vi "Render Energy.vi"(7 "Renderer":refnum<class "Renderer.lvclass">, 8 "error in (no error)":errorcluster, 11 "Ship in":refnum<class "Ship.lvclass">) -> (0 "error out":errorcluster)   [LabVIEW 2021, in "Ship.lvclass"]
uses:
  Ship.lvclass
  C:/dev/LabVIEW/LabMelee/Source/Application Specific/Element/Element.lvclass
  Renderer/Renderer.lvclass
  Element/Element.lvclass/Element.ctl
  Ship.lvclass/Ship.ctl
  Re-use Libraries/Vector 2D/Vector 2D.lvclass/Vector 2D.ctl
  Re-use Libraries/Vector 2D/Vector 2D.lvclass
  Element/Element.lvclass
  LabSDL2/Source/Libraries/LibSDL2 Wrapper/LibSDL2.lvlib
panel:
  in  "x Offset From Sidebar":i32=180
  in  "y Offset":i32=230
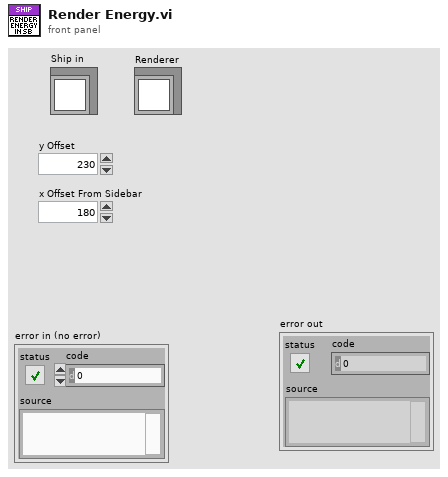
[diagram p1: front panel]
types:
  T1 = typedef "Constants.ctl" = cluster{"Colours":cluster{"OK":u32, "Warning":u32, "Error":u32, "Red":u32, "Green":u32, "Blue":u32, "Yellow":u32, "Health":u32, "Energy":u32}, "System":cluster{"Target Frames Second":dbl, "Windows Size":refnum<class "Vector 2D.lvclass">, "World Size":refnum<class "Vector 2D.lvclass">, "Battle Area Size":refnum<class "Vector 2D.lvclass">, "Sidebar Width":sgl, "SC2 Frame Rate [Seconds/Frame]":sgl, "Sidebar Player 2 Y Offset":sgl}, "Game":cluster{"Maximum Asteroids":i32, "Max Energy":i32, "Max Crew":i32, "Maximum Stars":i32}}
  T2 = typedef "Element.lvclass/Player Type.ctl" = enum16{"Neutral", "Player 1", "Player 2"}
  T3 = typedef "LibSDL2.lvlib/Rectangle.ctl" = cluster{"x":i32, "y":i32, "Width":i32, "Height":i32}
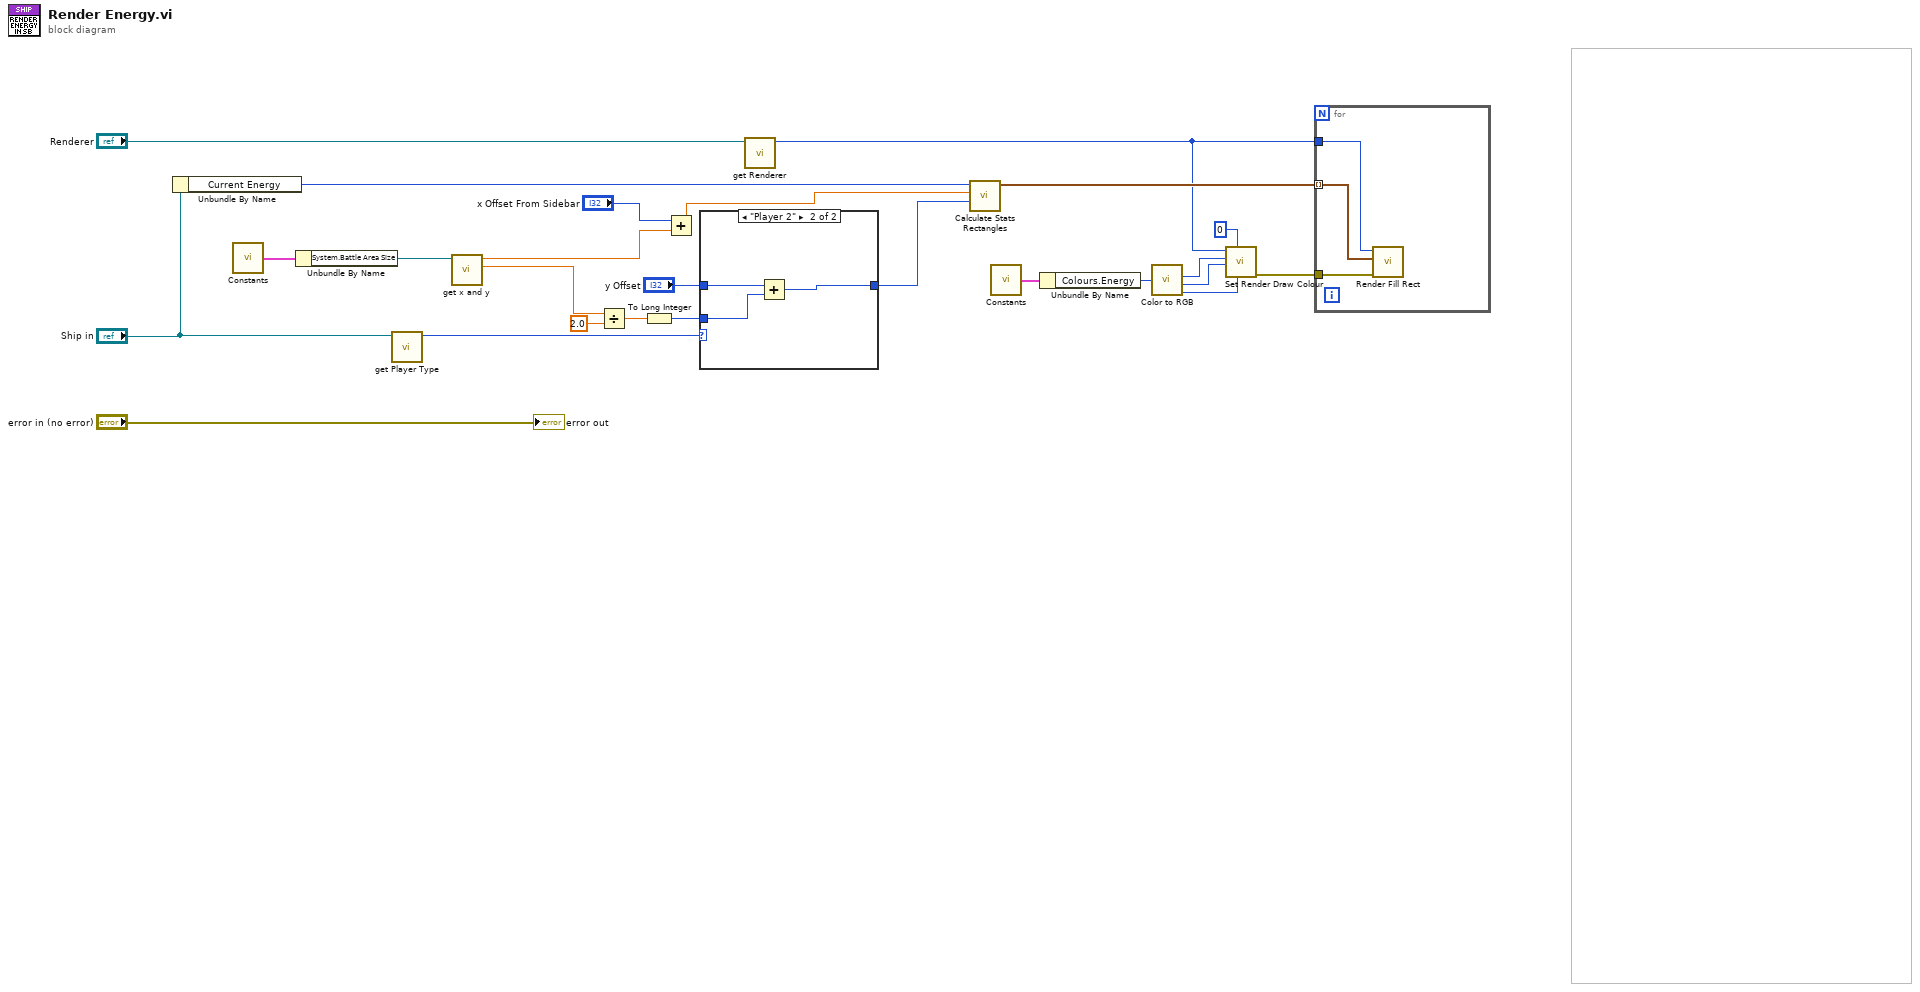
[diagram p0: block diagram]
diagram:
  n1 = Unbundle By Name("Ship in") -> ("Current Energy"=w14:i32)
  n2 = call "Constants.vi"() -> ("Constants"=w25:T1)
  n3 = Unbundle By Name(w25) -> ("System.Battle Area Size"=w10:refnum<class "Vector 2D.lvclass">)
  n4 = call "get Player Type.vi"("Element in"="Ship in") -> ("Player Type"=w24:T2)  [unwired: 10 in]
  n5 = call "get x and y.vi"("Vector 2D in"=w10) -> ("y"=w1:sgl, "x"=w4:sgl)  [unwired: 9 in]
  n6 = Divide(x=w1, y=sgl 2.0) -> (x/y=w6:sgl)
  n7 = To Long Integer(number=w6) -> (32bit integer=w5:i32)
  n8 = Add(x="x Offset From Sidebar", y=w4) -> (x+y=w2:sgl)
  n9 = case shown="\"Player 2\"" w24 {
    tunnel: [w26 w27] -> w7
    tunnel: "y Offset" -> [w26 w29]
    tunnel: w5 -> [_ w28]
    frame "Player 1", Default {
    }
    frame "Player 2" {
      n10 = Add(x=w29, y=w28) -> (x+y=w27:i32)
    }
  }
  n11 = call-dynamic "get Renderer.vi"("Renderer in"="Renderer") -> ("Renderer"=w12:u32)  [unwired: 10 in]
  n12 = call "Calculate Stats Rectangles.vi"("Start y"=w7, "Start x"=w2, "Count"=w14) -> ("Rectangles"=w13:T3[])  [unwired: 8 in]
  n13 = call "Constants.vi"() -> ("Constants"=w20:T1)
  n14 = Unbundle By Name(w20) -> ("Colours.Energy"=w18:u32)
  n15 = call <vilib>:"Color to RGB.vi"("Color"=w18) -> ("R"=w17:u8, "G"=w16:u8, "B"=w15:u8)  [unwired: 1 out]
  n16 = call "Set Render Draw Colour.vi"("B"=w15, "A"=u8 0, "G"=w16, "R"=w17, "Renderer Pointer"=w12) -> ("error out"=w11:errorcluster)  [unwired: 5 in, 1 out]
  n17 = for {
    tunnel: w13 -> [w31] mode=indexing
    tunnel: w12 -> [w32]
    tunnel: w11 -> [w30]
    n18 = call "Render Fill Rect.vi"("error in"=w30, "Rectangle"=w31, "Renderer Pointer"=w32) -> ()  [unwired: 7 in, 2 out]
  }
  "error out" <- "error in (no error)"
